vi "Get_motors_positions.vi"(8 "error in (no error)":errorcluster) -> (0 "m6":dbl, 1 "m5":dbl, 2 "m3":dbl, 3 "m2":dbl, 4 "error out":errorcluster)   [LabVIEW 2017]
uses:
  IP Address.vi
  <vilib>/httpClient/LabVIEWHTTPClient.lvlib
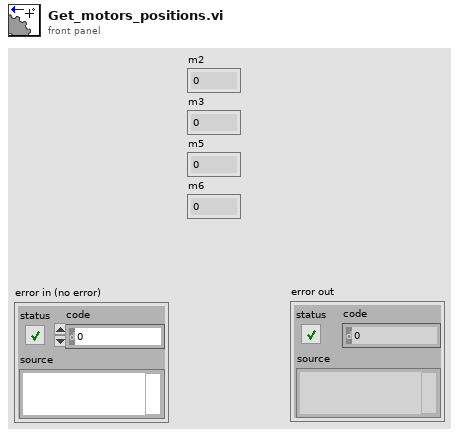
[diagram p1: front panel]
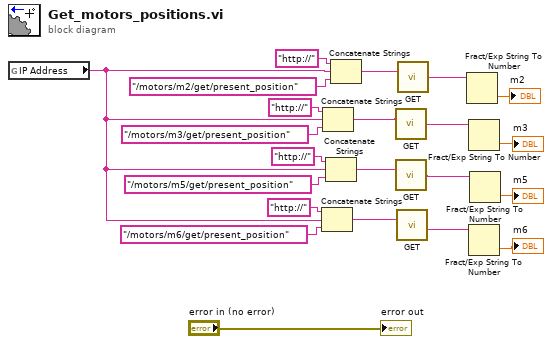
[diagram p0: block diagram]
diagram:
  n1 = global read "IP Address.vi" "IP Address"() -> (w1:string)
  n2 = Concatenate Strings("http://" ("string"), w1, "/motors/m6/get/present_position" ("url")) -> (w3:string)
  n3 = Concatenate Strings("http://" ("string"), w1, "/motors/m3/get/present_position" ("url")) -> (w5:string)
  n4 = Concatenate Strings("http://" ("string"), w1, "/motors/m5/get/present_position" ("url")) -> (w4:string)
  n5 = Concatenate Strings("http://" ("string"), w1, "/motors/m2/get/present_position" ("url")) -> (w11:string)
  n6 = call <vilib>:"GET.vi"("url"=w5) -> ("body"=w20:string)  [unwired: 11 in, 3 out]
  n7 = call <vilib>:"GET.vi"("url"=w4) -> ("body"=w21:string)  [unwired: 11 in, 3 out]
  n8 = call <vilib>:"GET.vi"("url"=w3) -> ("body"=w22:string)  [unwired: 11 in, 3 out]
  n9 = call <vilib>:"GET.vi"("url"=w11) -> ("body"=w19:string)  [unwired: 11 in, 3 out]
  n10 = Fract/Exp String To Number(string=w19) -> (number=→"m2":dbl)  [unwired: 3 in, 1 out]
  n11 = Fract/Exp String To Number(string=w20) -> (number=→"m3":dbl)  [unwired: 3 in, 1 out]
  n12 = Fract/Exp String To Number(string=w22) -> (number=→"m6":dbl)  [unwired: 3 in, 1 out]
  n13 = Fract/Exp String To Number(string=w21) -> (number=→"m5":dbl)  [unwired: 3 in, 1 out]
  "error out" <- "error in (no error)"
